vi "WPI_CameraManageConnections.vi"(4 "Cluster":T4, 7 "parameters":T2(array[cluster]), 8 "NT Connection":bool, 9 "Camera Name":string, 10 "Operation":enum16{"Read", "Reopen", "Close"}(ring), 11 "Refnum in":T1) -> (0 "error out":errorcluster, 2 "Active":bool, 3 "Refnum out":T1, 5 "Bandwidth (Mbps)":dbl)   [LabVIEW 2017]
uses:
  <vilib>/Rock Robotics/WPI/Camera/WPI_CameraImageSize.ctl
  <vilib>/vision/Image Controls.llb/IMAQ Image.ctl
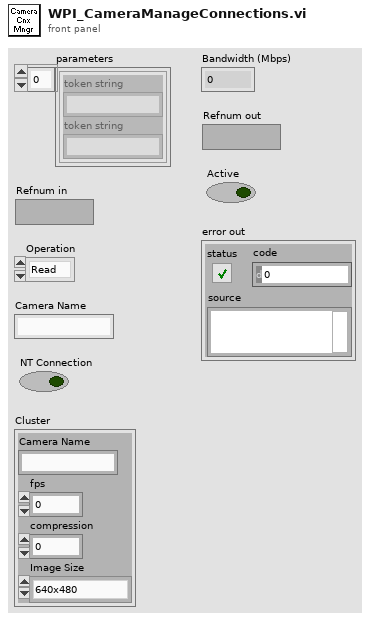
[diagram p1: front panel]
types:
  T1 = typedef "IMAQ Image.ctl" = refnum<image>
  T2 = cluster{"token string":string, "token string":string}[]
  T3 = typedef "WPI_CameraImageSize.ctl" = enum16{"640x480", "320x240", "160x120", "Custom"}
  T4 = cluster{"Camera Name":string, "fps":i32, "compression":i32, "Image Size":T3}
  T5 = cluster{"token string":string, "token string 2":string}[]
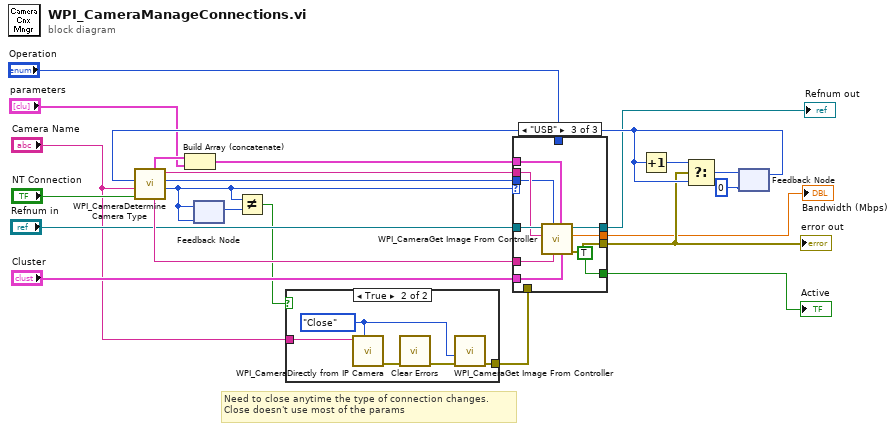
[diagram p0: block diagram]
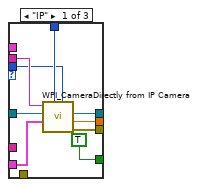
[diagram p3: hidden frame]
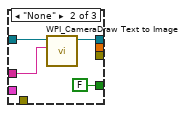
[diagram p4: hidden frame]
diagram:
  # "Need to close anytime the type of connection changes.\nClose doesn't use most of the params"
  n1 = feedback #1(0) -> (w21:i32)
  n2 = call <vilib>:"WPI_CameraDetermine Camera Type.vi"("NT Connection"="NT Connection", "Camera Name"="Camera Name", "iteration"=w21) -> ("Camera Type"=w6:enum16{"None", "USB", "IP"}, "port"=w13:i32, "address"=w1:string, "cgi string"=w14:string, "parameters"=w16:T5)  [unwired: 4 in]
  n3 = Build Array (concatenate)(w16, "parameters") -> (w15:T2)
  n4 = feedback-in #2(w6) -> ()
  n5 = feedback #2(w6) -> (w7:enum16{"None", "USB", "IP"})
  n6 = Not Equal?(x=w6, y=w7) -> (x != y?=w5:bool)
  n7 = case shown="True" w5 {
    tunnel: [_ w28] -> w4
    tunnel: "Camera Name" -> [_ w26]
    frame False {
    }
    frame True {
      w27 = enum16{"Read", "Reopen", "Close"}."Close" ("Operation")
      n8 = call <vilib>:"WPI_CameraDirectly from IP Camera.vi"("Operation"=w27, "address"=w26) -> ("error out"=w25:errorcluster)  [unwired: 7 in, 2 out]
      n9 = call <vilib>:"Clear Errors.vi"("error in (no error)"=w25) -> ("error out"=w24:errorcluster)  [unwired: 5 in, 1 out]
      n10 = call <vilib>:"WPI_CameraGet Image From Controller.vi"("error in (no error)"=w24, "Operation"=w27) -> ("error out"=w28:errorcluster)  [unwired: 7 in, 2 out]
    }
  }
  n11 = case shown="\"USB\"" w6 {
    tunnel: "Cluster" -> [w37 _ w47]
    tunnel: "Operation" -> [w31 _ _]
    tunnel: [w35 _ w46] -> w9
    tunnel: "Refnum in" -> [w33 w39 w51]
    tunnel: w1 -> [w32 _ w48]
    tunnel: [w36 _ w49] -> w18
    tunnel: [w34 w40 w50] -> w11
    tunnel: [TRUE FALSE TRUE] -> w12
    tunnel: w13 -> [w29 _ w44]
    tunnel: w14 -> [_ w38 w43]
    tunnel: w15 -> [_ _ w42]
    tunnel: w4 -> [_ _ _]
    frame "IP" {
      n12 = call <vilib>:"WPI_CameraDirectly from IP Camera.vi"("port"=w29, "Operation"=w31, "Camera Settings"=w37, "Image"=w33, "address"=w32) -> ("error out"=w36:errorcluster, "Bandwidth (Mbps)"=w35:dbl, "Image Out"=w34:T1)  [unwired: 4 in]
    }
    frame "None" {
      n13 = call <vilib>:"WPI_CameraDraw Text to Image.vi"("Text"=w38, "Refnum in"=w39) -> ("Refnum out"=w40:T1)  [unwired: 9 in]
    }
    frame "USB" {
      n14 = call <vilib>:"WPI_CameraGet Image From Controller.vi"("Camera Settings"=w47, "parameters"=w42, "cgi String"=w43, "port"=w44, "Controller Address"=w48, "Image"=w51) -> ("error out"=w49:errorcluster, "Bandwidth (Mbps)"=w46:dbl, "Image Out"=w50:T1)  [unwired: 3 in]
    }
  }
  "error out" <- w18
  "Active" <- w12
  "Refnum out" <- w11
  "Bandwidth (Mbps)" <- w9
  n15 = Increment(x=w21) -> (x+1=w19:i32)
  n16 = Select(t=w19, s=w18, f=w21) -> (s? t:f=w20:i32)
  n17 = feedback-in #1(w20) -> ()
